vi "Bristol_WM_SA_ver2.vi"() -> ()   [LabVIEW 2012]
uses:
  <vilib>/DAQmx/write.llb/DAQmx Write (Digital 1D Bool NChan 1Samp 1Line).vi
  <vilib>/DAQmx/miscellaneous.llb/DAQmx Fill In Error Info.vi
panel:
  in  "HSRL_WV":bool
  in  "TimeOut":i32=1000
  in  "WV_On/Off":bool
  in  "stop":bool
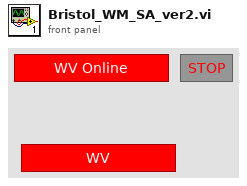
[diagram p1: front panel]
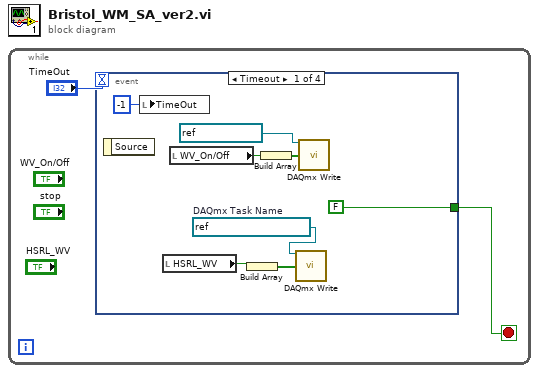
[diagram p0: block diagram]
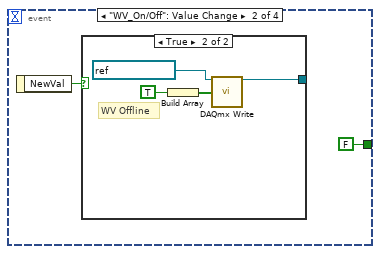
[diagram p2: hidden frame]
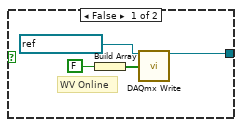
[diagram p3: hidden frame]
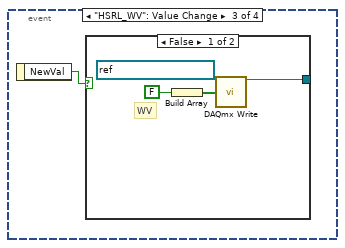
[diagram p4: hidden frame]
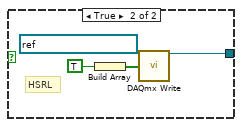
[diagram p5: hidden frame]
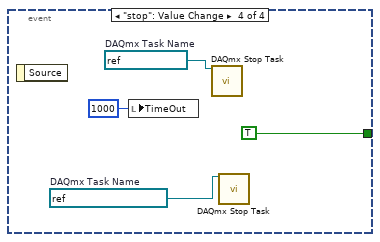
[diagram p6: hidden frame]
diagram:
  n1 = while {
    stop <- w2 stop-if-true
    n2 = event shown="[0] Timeout" {
      selector: _ -> [_ _ _ _]
      dyn-events: _ -> [_ _ _ _]
      timeout: "TimeOut" -> [_ _ _ _]
      tunnel: [FALSE ("Boolean") FALSE ("Boolean") _ TRUE ("Boolean")] -> w2
      event Timeout {
        w3 = refnum<k21> "HSRL_WV_switch"  # DAQmx Task Name
        n3 = event-data() -> ()  [unwired: 1 in, 1 out]
        n4 = local write "TimeOut"(-1 ("TimeOut")) -> ()
        n5 = local read "HSRL_WV"() -> (w5:bool)
        n6 = local read "WV_On/Off"() -> (w6:bool)
        n7 = Build Array(w5) -> (w4:bool[])
        n8 = Build Array(w6) -> (w7:bool[])
        n9 = call-poly <vilib>:"DAQmx Write.vi"("task/channels in"=w3, "data"=w4) -> ()  [unwired: 11 in, 3 out]
        n10 = call-poly <vilib>:"DAQmx Write.vi"("task/channels in"=refnum<k21> "BristolWM", "data"=w7) -> ()  [unwired: 11 in, 3 out]
      }
      event "WV_On/Off": Value Change {
        n11 = event-data() -> ("NewVal"=w12:bool)  [unwired: 1 in]
        n12 = case shown="True" w12 {
          tunnel: [w15 w19] -> _
          frame False {
            # "WV Online"
            n13 = Build Array(FALSE ("Boolean")) -> (w13:bool[])
            n14 = call-poly <vilib>:"DAQmx Write.vi"("task/channels in"=refnum<k21> "BristolWM", "data"=w13) -> ("task out"=w15:refnum<k21>)  [unwired: 11 in, 2 out]
          }
          frame True {
            # "WV Offline"
            n15 = Build Array(TRUE ("Boolean")) -> (w17:bool[])
            n16 = call-poly <vilib>:"DAQmx Write.vi"("task/channels in"=refnum<k21> "BristolWM", "data"=w17) -> ("task out"=w19:refnum<k21>)  [unwired: 11 in, 2 out]
          }
        }
      }
      event "HSRL_WV": Value Change {
        n17 = event-data() -> ("NewVal"=w21:bool)  [unwired: 1 in]
        n18 = case shown="False" w21 {
          tunnel: [w24 w28] -> _
          frame False {
            # "WV"
            n19 = Build Array(FALSE ("Boolean")) -> (w22:bool[])
            n20 = call-poly <vilib>:"DAQmx Write.vi"("task/channels in"=refnum<k21> "HSRL_WV_switch", "data"=w22) -> ("task out"=w24:refnum<k21>)  [unwired: 11 in, 2 out]
          }
          frame True {
            # "HSRL"
            n21 = Build Array(TRUE ("Boolean")) -> (w26:bool[])
            n22 = call-poly <vilib>:"DAQmx Write.vi"("task/channels in"=refnum<k21> "HSRL_WV_switch", "data"=w26) -> ("task out"=w28:refnum<k21>)  [unwired: 11 in, 2 out]
          }
        }
      }
      event "stop": Value Change {
        w30 = refnum<k21> "BristolWM"  # DAQmx Task Name
        w31 = refnum<k21> "HSRL_WV_switch"  # DAQmx Task Name
        n23 = event-data() -> ()  [unwired: 1 in, 1 out]
        n24 = local write "TimeOut"(1000 ("TimeOut")) -> ()
        n25 = call <vilib>:"DAQmx Stop Task.vi"("task/channels in"=w30) -> ()  [unwired: 13 in, 2 out]
        n26 = call <vilib>:"DAQmx Stop Task.vi"("task/channels in"=w31) -> ()  [unwired: 13 in, 2 out]
      }
    }
  }
